vi "Checksum.vi"(10 "Checksum (Off)":bool, 11 "Input":string) -> (2 "Data Buffer":string, 3 "Checksum Pass?":bool)   [LabVIEW 2014, in "Hokuyo URG Series.lvlib"]
doc: "This VI does checksumming in SCIP 2.0. When 'Checksum' is turned on, the boolean \"Checksum Pass?\" indicates if the input buffer passed or failed the checksum.\n\nRegardless of whether or not the 'Checksum' is on this VI strips the input buffer of the trailing newline and checksum byte."
uses:
  Hokuyo URG Series.lvlib
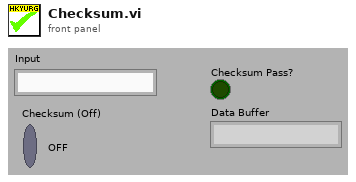
[diagram p1: front panel]
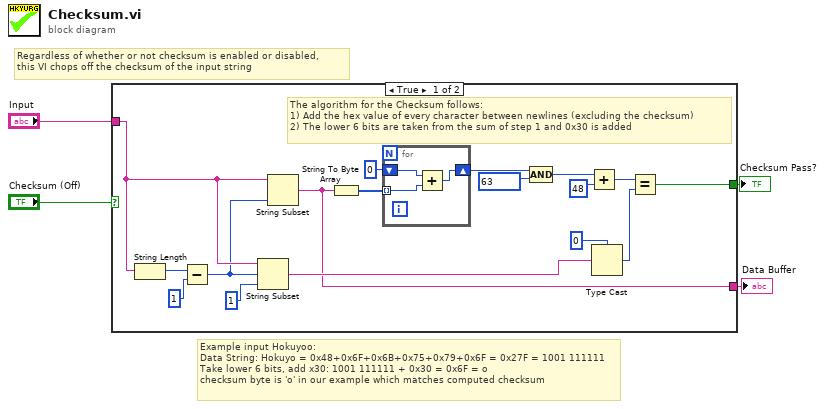
[diagram p0: block diagram]
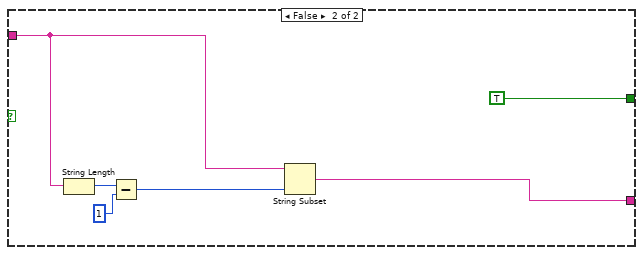
[diagram p2: hidden frame]
diagram:
  # "Regardless of whether or not checksum is enabled or disabled, \nthis VI chops off the checksum of the input string"
  # "Example input Hokuyoo:\nData String: Hokuyo = 0x48+0x6F+0x6B+0x75+0x79+0x6F = 0x27F = 1001 111111\nTake lower 6 bits, add x30: 1001 111111 + 0x30 = 0x6F = o\nchecksum byte is 'o' in our example which matches computed checksum"
  n1 = case shown="True" "Checksum (Off)" {
    tunnel: [w11 TRUE] -> w4
    tunnel: "Input" -> [w10 w28]
    tunnel: [w8 w26] -> w2
    frame True {
      # "The algorithm for the Checksum follows:\n1) Add the hex value of every character between newlines (excluding the checksum)\n2) The lower 6 bits are taken from the sum of step 1 and 0x30 is added"
      n2 = String Length(string=w10) -> (length=w17:i32)
      n3 = Subtract(x=w17, y=1) -> (x-y=w9:i32)
      n4 = String Subset(string=w10, offset (0)=w9, length (rest)=1 ("length (rest)")) -> (substring=w14:string)
      n5 = String Subset(string=w10, length (rest)=w9) -> (substring=w8:string)  [unwired: 1 out]
      n6 = String To Byte Array(string=w8) -> (unsigned byte array=w20:u8[])
      n7 = for {
        shift-right: [w22] -> w6
        shift-left: u32 0 -> [w24]
        tunnel: w20 -> [w23] mode=indexing
        n8 = Add(x=w24, y=w23) -> (x+y=w22:u32)
      }
      n9 = Compound Arithmetic op=AND(w6, u32 63 ("y")) -> (w5:u32)
      n10 = Add(x=w5, y=u32 48) -> (x+y=w13:u32)
      n11 = Type Cast(type=u8 0, x=w14) -> (*(type *) &x=w12:u8)
      n12 = Equal?(x=w13, y=w12) -> (x = y?=w11:bool)
    }
    frame False {
      n13 = String Length(string=w28) -> (length=w30:i32)
      n14 = Subtract(x=w30, y=1) -> (x-y=w27:i32)
      n15 = String Subset(string=w28, length (rest)=w27) -> (substring=w26:string)  [unwired: 1 out]
    }
  }
  "Checksum Pass?" <- w4
  "Data Buffer" <- w2
